vi "testPhasePlotting_modulo.vi"() -> ()   [LabVIEW 2025]
uses:
  <vilib>/measure/NI_MAPro.lvlib
panel:
  in  "Sampling info":cluster{"Fs":dbl, "#s":dbl}={"Fs"=10000.0, "#s"=1000.0} {"Fs" format="%.2p"}
  out "Frequency waveform":dynamicdata(graph)
  in  "stop":bool
  in  "Phase Unit":u16(ring) items=["Degree", "Radian"]
  out "Nominal Frequency unit (Hz)":string="Hz"
  out "Frequency unit (Hz)":string="Hz"
  out "Phase unit (deg)":string="deg"
  out "Phase  unit (rad)":string="rad"
  in  "Nominal Frequency":dbl=50.0
  in  "Frequency":dbl=50.0
  in  "Phase":dbl
  out "Phase waveform":waveform(dbl)(graph)
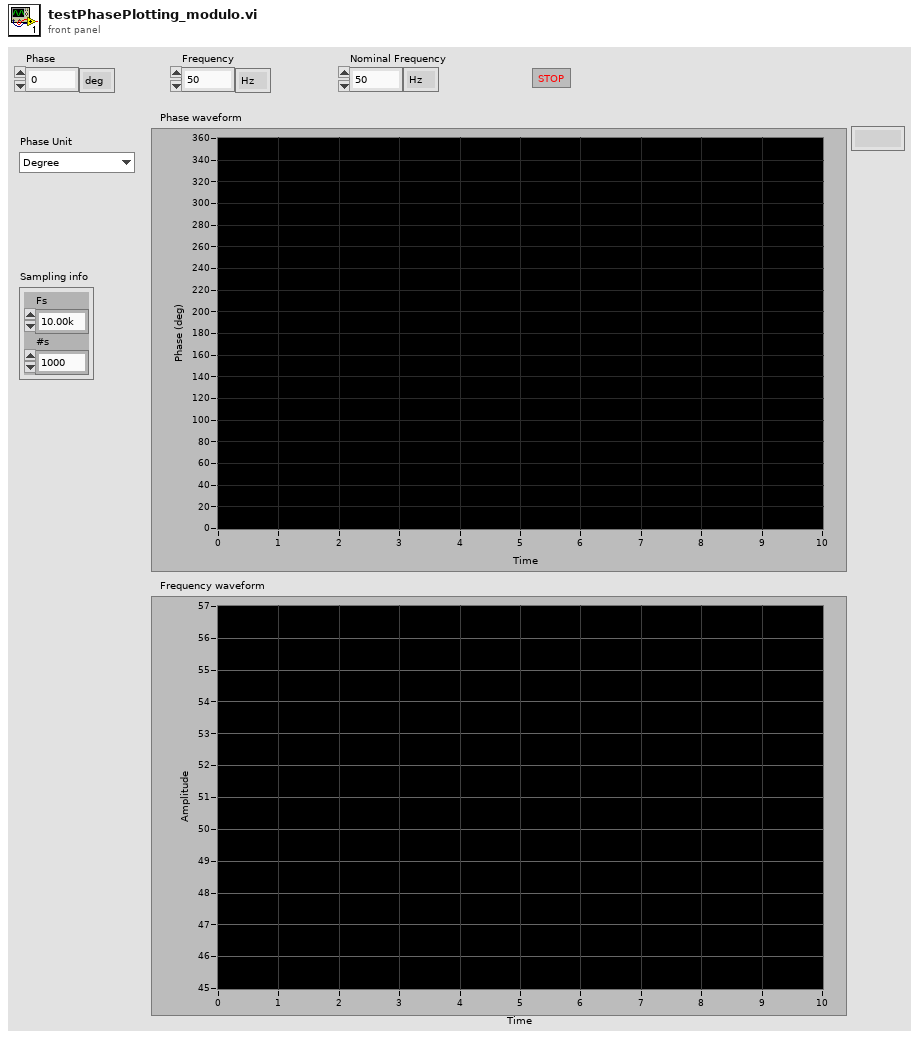
[diagram p1: front panel]
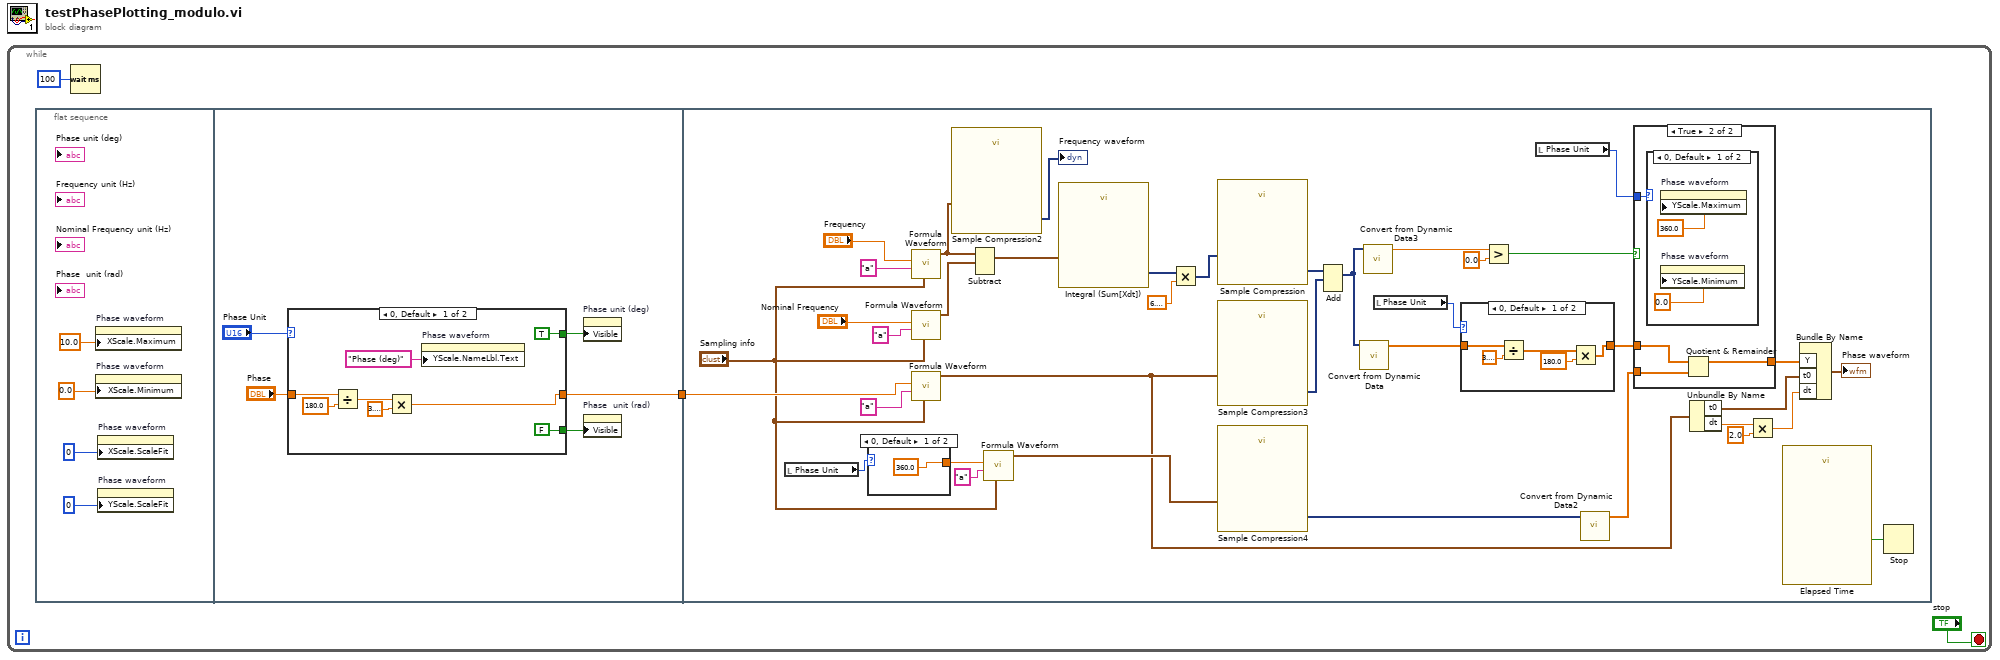
[diagram p0: block diagram]
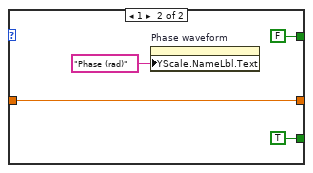
[diagram p2: hidden frame]
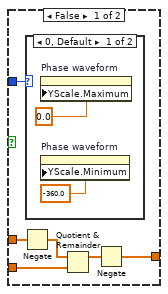
[diagram p3: hidden frame]
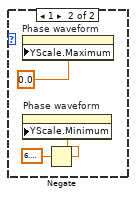
[diagram p4: hidden frame]
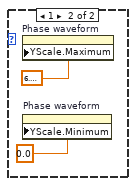
[diagram p5: hidden frame]
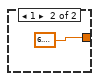
[diagram p6: hidden frame]
diagram:
  n1 = while {
    stop <- "stop" stop-if-true
    n2 = flat-sequence {
      tunnel: [w9] -> w3
      tunnel: w3 -> [w60]
      frame #0 {
        n3 = property on="Phase waveform" class="WFChart (strict)"("XScale.Maximum"=10.0 ("X Scale.Range:Maximum")) -> ()  [unwired: 2 in, 2 out]
        n4 = property on="Phase waveform" class="WFChart (strict)"("XScale.Minimum"=0.0 ("X Scale.Range:Minimum")) -> ()  [unwired: 2 in, 2 out]
        n5 = property on="Phase waveform" class="WFChart (strict)"("XScale.ScaleFit"=u8 0 ("X Scale.Scale Fit")) -> ()  [unwired: 2 in, 2 out]
        n6 = property on="Phase waveform" class="WFChart (strict)"("YScale.ScaleFit"=u8 0 ("Y Scale.Scale Fit")) -> ()  [unwired: 2 in, 2 out]
      }
      frame #1 {
        n7 = case shown="0, Default" "Phase Unit" {
          tunnel: [TRUE FALSE] -> w12
          tunnel: [FALSE TRUE] -> w11
          tunnel: "Phase" -> [w16 w21]
          tunnel: [w13 w21] -> w9
          frame 0, Default {
            n8 = Divide(x=w16, y=180.0) -> (x/y=w15:dbl)
            n9 = Multiply(x=w15, y=3.141592653589793) -> (x*y=w13:dbl)
            n10 = property on="Phase waveform" class="WFChart (strict)"("YScale.NameLbl.Text"="Phase (deg)" ("Y Scale.Name Label.Text")) -> ()  [unwired: 2 in, 2 out]
          }
          frame 1 {
            n11 = property on="Phase waveform" class="WFChart (strict)"("YScale.NameLbl.Text"="Phase (rad)" ("Y Scale.Name Label.Text")) -> ()  [unwired: 2 in, 2 out]
          }
        }
        n12 = property on="Phase unit (deg)" class="Str"("Visible"=w12) -> ()  [unwired: 2 in, 2 out]
        n13 = property on="Phase  unit (rad)" class="Str"("Visible"=w11) -> ()  [unwired: 2 in, 2 out]
      }
      frame #2 {
        n14 = local read "Phase Unit"() -> (w43:u16)
        n15 = case shown="0, Default" w43 {
          tunnel: [360.0 6.283185307179586] -> w42
          frame 0, Default {
          }
          frame 1 {
          }
        }
        n16 = call <vilib>:"Formula Waveform.vi"("sampling info"="Sampling info", "formula"="a", "amplitude"="Frequency") -> ("signal out"=w50:waveform(dbl))  [unwired: 7 in, 1 out]
        n17 = call <vilib>:"Formula Waveform.vi"("sampling info"="Sampling info", "formula"="a", "amplitude"="Nominal Frequency") -> ("signal out"=w49:waveform(dbl))  [unwired: 7 in, 1 out]
        n18 = call <vilib>:"Formula Waveform.vi"("sampling info"="Sampling info", "formula"="a", "amplitude"=w60) -> ("signal out"=w33:waveform(dbl))  [unwired: 7 in, 1 out]
        n19 = call "Sample Compression2"("Signals"=w50) -> ("Maximum"=→"Frequency waveform":dynamicdata)  [unwired: 8 in, 2 out]
        n20 = Subtract(1:w49, 2:w50) -> (0:w48:waveform(dbl))  [unwired: 1 in, 1 out]
        n21 = call <vilib>:"Formula Waveform.vi"("sampling info"="Sampling info", "formula"="a", "amplitude"=w42) -> ("signal out"=w44:waveform(dbl))  [unwired: 7 in, 1 out]
        n22 = call "Integral (Sum[Xdt])"("Signals"=w48) -> ("Result"=w52:dynamicdata)  [unwired: 5 in, 1 out]
        n23 = Multiply(x=w52, y=6.283185307179586) -> (x*y=w54:dynamicdata)
        n24 = call "Sample Compression"("Signals"=w54) -> ("Maximum"=w53:dynamicdata)  [unwired: 8 in, 2 out]
        n25 = call "Sample Compression3"("Signals"=w33) -> ("Maximum"=w37:dynamicdata)  [unwired: 8 in, 2 out]
        n26 = call "Sample Compression4"("Signals"=w44) -> ("Maximum"=w34:dynamicdata)  [unwired: 8 in, 2 out]
        n27 = Add(1:w37, 2:w53) -> (0:w28:dynamicdata)  [unwired: 1 in, 1 out]
        n28 = call "Convert from Dynamic Data"("Dynamic Data Type"=w28) -> ("Array"=w40:dbl[])  [unwired: 3 in]
        n29 = call "Convert from Dynamic Data3"("Dynamic Data Type"=w28) -> ("Scalar"=w27:dbl)  [unwired: 3 in]
        n30 = local read "Phase Unit"() -> (w55:u16)
        n31 = case shown="0, Default" w55 {
          tunnel: w40 -> [w88 w89]
          tunnel: [w85 w89] -> w41
          frame 0, Default {
            n32 = Divide(x=w88, y=3.141592653589793) -> (x/y=w87:dbl[])
            n33 = Multiply(x=w87, y=180.0) -> (x*y=w85:dbl[])
          }
          frame 1 {
          }
        }
        n34 = Greater?(x=w27, y=0.0) -> (0:w38:bool)
        n35 = local read "Phase Unit"() -> (w26:u16)
        n36 = call "Convert from Dynamic Data2"("Dynamic Data Type"=w34) -> ("Array"=w39:dbl[])  [unwired: 3 in]
        n37 = case shown="True" w38 {
          tunnel: w41 -> [w67 w77]
          tunnel: w39 -> [w66 w76]
          tunnel: [w65 w75] -> w36
          tunnel: w26 -> [w63 w74]
          frame False {
            n38 = Negate(x=w67) -> (-x=w68:dbl[])
            n39 = case shown="0, Default" w63 {
              frame 0, Default {
                n40 = property on="Phase waveform" class="WFChart (strict)"("YScale.Maximum"=0.0 ("Y Scale.Range:Maximum")) -> ()  [unwired: 2 in, 2 out]
                n41 = property on="Phase waveform" class="WFChart (strict)"("YScale.Minimum"=-360.0 ("Y Scale.Range:Minimum")) -> ()  [unwired: 2 in, 2 out]
              }
              frame 1 {
                n42 = property on="Phase waveform" class="WFChart (strict)"("YScale.Maximum"=0.0 ("Y Scale.Range:Minimum")) -> ()  [unwired: 2 in, 2 out]
                n43 = Negate(x=6.283185307179586) -> (-x=w71:dbl)
                n44 = property on="Phase waveform" class="WFChart (strict)"("YScale.Minimum"=w71) -> ()  [unwired: 2 in, 2 out]
              }
            }
            n45 = Quotient & Remainder(x=w68, y=w66) -> (x-y*floor(x/y)=w64:dbl[])  [unwired: 1 out]
            n46 = Negate(x=w64) -> (-x=w65:dbl[])
          }
          frame True {
            n47 = case shown="0, Default" w74 {
              frame 0, Default {
                n48 = property on="Phase waveform" class="WFChart (strict)"("YScale.Maximum"=360.0 ("Y Scale.Range:Maximum")) -> ()  [unwired: 2 in, 2 out]
                n49 = property on="Phase waveform" class="WFChart (strict)"("YScale.Minimum"=0.0 ("Y Scale.Range:Minimum")) -> ()  [unwired: 2 in, 2 out]
              }
              frame 1 {
                n50 = property on="Phase waveform" class="WFChart (strict)"("YScale.Maximum"=6.283185307179586) -> ()  [unwired: 2 in, 2 out]
                n51 = property on="Phase waveform" class="WFChart (strict)"("YScale.Minimum"=0.0 ("Y Scale.Range:Minimum")) -> ()  [unwired: 2 in, 2 out]
              }
            }
            n52 = Quotient & Remainder(x=w77, y=w76) -> (x-y*floor(x/y)=w75:dbl[])  [unwired: 1 out]
          }
        }
        n53 = Unbundle By Name(w33) -> ("t0"=w32:timestamp, "dt"=w31:dbl)
        n54 = Multiply(x=w31, y=2.0) -> (x*y=w30:dbl)
        n55 = call "Elapsed Time"() -> ("Time has Elapsed"=w25:bool)  [unwired: 12 in, 7 out]
        n56 = Bundle By Name("Y"=w36, "t0"=w32, "dt"=w30) -> (→"Phase waveform":waveform(dbl))  [unwired: 1 in]
        n57 = Stop(stop? (T)=w25) -> ()
      }
    }
    n58 = Wait (ms)(milliseconds to wait=u32 100) -> ()  [unwired: 1 out]
  }
